vi "dfd_DFXPSimu SymAdd (ss).vi"(5 "quantize output? (T)":bool=TRUE, 7 "op params":T2={"source"=0, "is floating?"=FALSE, "o-mode"=enum."Wrap", "q-mode"=enum."Truncation", "wl"=1, "high limit"=0, "low limit"=0, "iwl"=0, "sign?"=TRUE} {"source" items=["Coef a/k"=0, "Coef b/v"=7, "Input"=1, "Output"=2, "Multiplicand"=3, "Product"=4, "Sum"=5, "Delay"=6, "Gain"=8]}, 8 "filtering statistics in":T6(array[cluster]) {"statistics information"."min value" format="%.2f"; "statistics information"."max value" format="%.2f"; "Quantizer Source" items=["Coefficients a/k"=0, "Coefficients b/v"=7, "Input"=1, "Output"=2, "Multiplicand"=3, "Product"=4, "Sum"=5, "Delay"=6]}, 10 "value in 2":T1={"value"=0, "wl"=0, "iwl"=0, "Signed"=TRUE} {"value" format="%.0x"}, 11 "value in 1":T1={"value"=0, "wl"=0, "iwl"=0, "Signed"=TRUE} {"value" format="%.0x"}) -> (0 "filtering statistics out":T6(array[cluster]) {"statistics information"."min value" format="%.2f"; "statistics information"."max value" format="%.2f"; "Quantizer Source" items=["Coefficients a/k"=0, "Coefficients b/v"=7, "Input"=1, "Output"=2, "Multiplicand"=3, "Product"=4, "Sum"=5, "Delay"=6]}, 3 "value out":T1={"value"=0, "wl"=0, "iwl"=0, "Signed"=TRUE} {"value" format="%.0x"})   [LabVIEW 2017, in "NI_DigFilter_FXP.lvlib"]
uses:
  <vilib>/addons/Digital Filter Design/NI_DigFilter_FXP.lvlib
  <vilib>/addons/Digital Filter Design/_Objects.llb/dfd_DFXP Data Type (scaler).ctl
  <vilib>/addons/Digital Filter Design/_Objects.llb/DFD Quantization Sources.ctl
  <vilib>/addons/Digital Filter Design/_Objects.llb/DFD FXP Statistics Data.ctl
  <vilib>/addons/Digital Filter Design/_Objects.llb/dfd_DFXP Operation Parameter.ctl
  <vilib>/addons/Digital Filter Design/_Objects.llb/dfd_Internal Quantization Srcs.ctl
  <vilib>/addons/Digital Filter Design/NI_DigFilterLicensed.lvlib
panel:
  in  "Value type":T1={"value"=0, "wl"=0, "iwl"=0, "Signed"=TRUE} {"value" format="%.0x"}
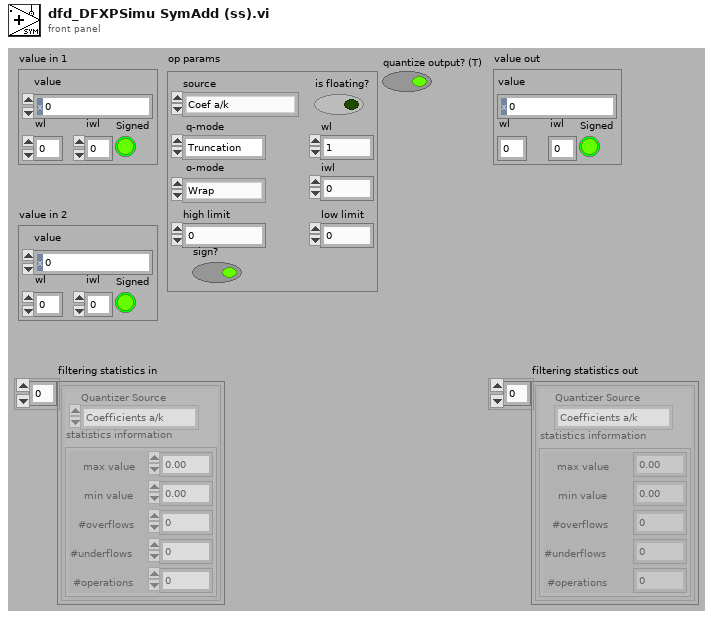
[diagram p1: front panel]
types:
  T1 = typedef "dfd_DFXP Data Type (scaler).ctl" = cluster{"value":i64, "wl":i16, "iwl":i16, "Signed":bool}
  T2 = typedef "dfd_DFXP Operation Parameter.ctl" = cluster{"source":T3, "is floating?":bool, "o-mode":enum16{"Saturation", "Wrap"}, "q-mode":enum16{"Nearest", "Truncation"}, "wl":i16, "high limit":i64, "low limit":i64, "iwl":i16, "sign?":bool}
  T3 = typedef "NI_DigFilterLicensed.lvlib/dfd_Internal Quantization Srcs.ctl" = u16
  T4 = typedef "NI_DigFilterLicensed.lvlib/DFD Quantization Sources.ctl" = u16
  T5 = typedef "NI_DigFilterLicensed.lvlib/DFD FXP Statistics Data.ctl" = cluster{"max value":ext, "min value":ext, "#overflows":i32, "#underflows":i32, "#operations":i32}
  T6 = cluster{"Quantizer Source":T4, "statistics information":T5}[]
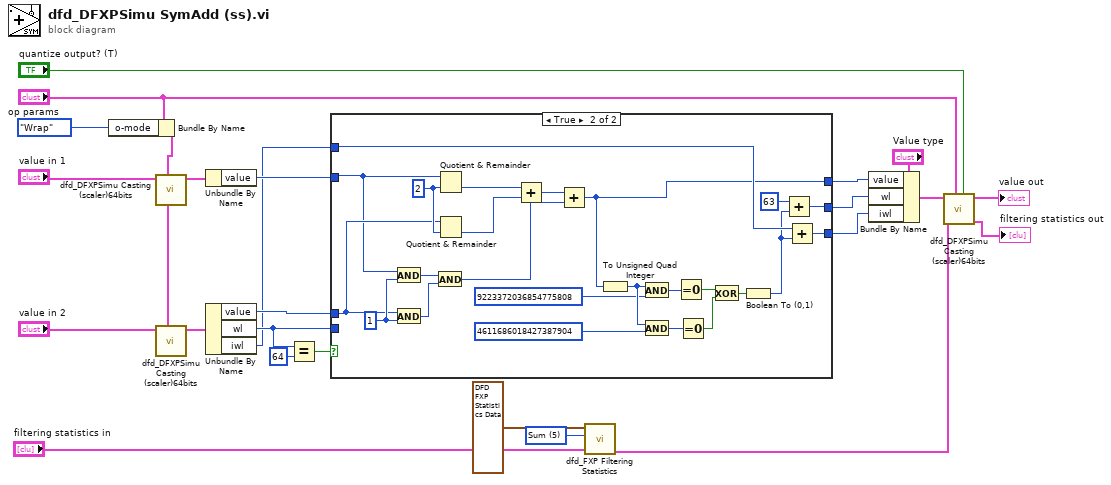
[diagram p0: block diagram]
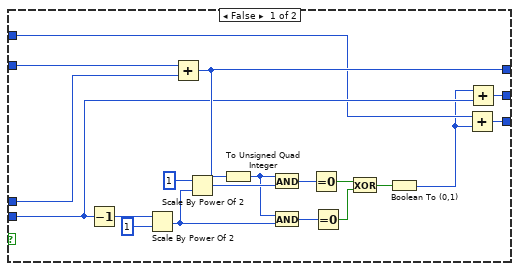
[diagram p2: hidden frame]
diagram:
  w4 = T3 5 items=["Coef a/k"=0, "Coef b/v"=7, "Input"=1, "Output"=2, "Multiplicand"=3, "Product"=4, "Sum"=5, "Delay"=6, "Gain"=8] ("source")
  n1 = Bundle By Name(cluster="op params", "o-mode"=enum16{"Saturation", "Wrap"}."Wrap" ("o_mode")) -> (w22:T2)
  n2 = call <vilib>:"dfd_DFXPSimu Casting (scaler)64bits.vi"("op params"=w22, "Value in"="value in 1") -> ("Value out"=w17:T1)  [unwired: 2 in, 7 out]
  n3 = call <vilib>:"dfd_DFXPSimu Casting (scaler)64bits.vi"("op params"=w22, "Value in"="value in 2") -> ("Value out"=w19:T1)  [unwired: 2 in, 7 out]
  n4 = Unbundle By Name(w17) -> ("value"=w16:i64)
  n5 = Unbundle By Name(w19) -> ("value"=w18:i64, "wl"=w8:i16, "iwl"=w5:i16)
  n6 = Equal?(x=w8, y=i16 64) -> (x = y?=w11:bool)
  n7 = case shown="True" w11 {
    tunnel: w16 -> [w44 w56]
    tunnel: w18 -> [w43 w57]
    tunnel: w8 -> [w37 _]
    tunnel: [w40 w61] -> w13
    tunnel: [w39 w65] -> w14
    tunnel: [w38 w46] -> w12
    tunnel: w5 -> [w36 w63]
    frame False {
      n8 = Decrement(x=w37) -> (x-1=w42:i16)
      n9 = Scale By Power Of 2(n=w42, x=u64 1) -> (x*2^n=w27:u64)
      n10 = Add(x=w44, y=w43) -> (x+y=w38:i64)
      n11 = Scale By Power Of 2(n=1 ("x"), x=w27) -> (x*2^n=w29:u64)
      n12 = To Unsigned Quad Integer(1:w38) -> (0:w28:u64)
      n13 = And(x=w28, y=w29) -> (x .and. y?=w32:u64)
      n14 = And(x=w28, y=w27) -> (x .and. y?=w31:u64)
      n15 = Equal To 0?(x=w32) -> (x = 0?=w34:bool)
      n16 = Equal To 0?(x=w31) -> (x = 0?=w33:bool)
      n17 = Exclusive Or(1:w33, 2:w34) -> (0:w30:bool)
      n18 = Boolean To (0,1)(Boolean=w30) -> (0, 1=w26:i16)
      n19 = Add(x=w36, y=w26) -> (x+y=w39:i16)
      n20 = Add(x=w26, y=w37) -> (x+y=w40:i16)
    }
    frame True {
      w58 = i64 1 ("y")
      w66 = i64 2 ("y")
      n21 = And(x=w56, y=w58) -> (x .and. y?=w60:i64)
      n22 = And(x=w57, y=w58) -> (x .and. y?=w59:i64)
      n23 = And(x=w60, y=w59) -> (x .and. y?=w55:i64)
      n24 = Quotient & Remainder(x=w56, y=w66) -> (floor(x/y)=w64:i64)  [unwired: 1 out]
      n25 = Quotient & Remainder(x=w57, y=w66) -> (floor(x/y)=w67:i64)  [unwired: 1 out]
      n26 = Add(x=w64, y=w67) -> (x+y=w68:i64)
      n27 = Add(x=w68, y=w55) -> (x+y=w46:i64)
      n28 = To Unsigned Quad Integer(1:w46) -> (0:w54:u64)
      n29 = And(x=w54, y=u64 9223372036854775808 ("x*2^n")) -> (x .and. y?=w52:u64)
      n30 = And(x=w54, y=u64 4611686018427387904 ("x*2^n")) -> (x .and. y?=w51:u64)
      n31 = Equal To 0?(x=w52) -> (x = 0?=w50:bool)
      n32 = Equal To 0?(x=w51) -> (x = 0?=w49:bool)
      n33 = Exclusive Or(1:w49, 2:w50) -> (0:w53:bool)
      n34 = Boolean To (0,1)(Boolean=w53) -> (0, 1=w45:i16)
      n35 = Add(x=i16 63, y=w45) -> (x+y=w61:i16)
      n36 = Add(x=w63, y=w45) -> (x+y=w65:i16)
    }
  }
  n37 = call <vilib>:"dfd_FXP Filtering Statistics.vi"("filtering statistics in"="filtering statistics in", "source"=w4, "new data"=T5 {"max value"=-inf, "min value"=inf, "#overflows"=0, "#underflows"=0, "#operations"=1}) -> ("filtering statistics out"=w1:T6)  [unwired: 8 out]
  n38 = Bundle By Name(cluster="Value type", "value"=w12, "wl"=w13, "iwl"=w14) -> (w9:T1)
  n39 = call <vilib>:"dfd_DFXPSimu Casting (scaler)64bits.vi"("quantize output?(T)"="quantize output? (T)", "op params"="op params", "filtering statistics in"=w1, "Value in"=w9) -> ("filtering statistics out"=→"filtering statistics out":T6, "Value out"=→"value out":T1)  [unwired: 6 out]
